vi "TDK_MsgManage.vi"(5 "CMD Type":T2=enum."SetADR", 6 "OUT?":bool, 7 "TDK Type":T1=enum."ZUP20-40", 8 "error in (no error)":errorcluster caption="error in", 9 "Current":dbl, 10 "Voltage":dbl, 11 "VISA resource name":refnum<visa-resource-name>) -> (0 "error out":errorcluster, 1 "Received Message":string, 3 "VISA resource name":refnum<visa-resource-name>, 4 "Serial Settings:Number of Bytes at Serial Port":u32)   [LabVIEW 2018]
uses:
  Def Ctrl/CMD Type.ctl
  Def Ctrl/TDK Type.ctl
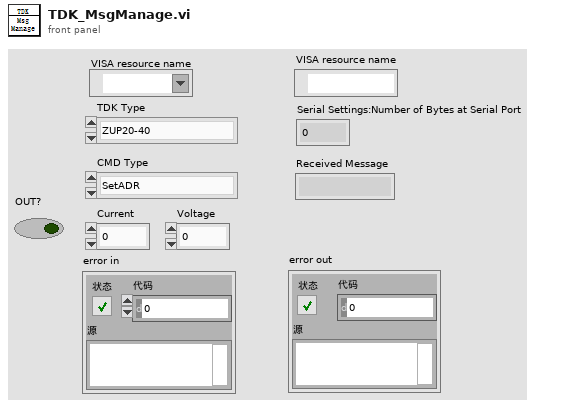
[diagram p1: front panel]
types:
  T1 = typedef "TDK Type.ctl" = enum16{"Default", "ZUP20-40", "Z+"}
  T2 = typedef "CMD Type.ctl" = enum16{"Default", "SetADR", "SetRMT", "SetVOL", "SetCUR", "SetOUT", "CheckREV", "CheckRMT", "CheckVOL", "CkeckCUR", "CheckOUT"}
  T3 = typedef "PowerSupplyCMD.ctl" = cluster{"ZUP20-40_CMD":T4, "Z+_CMD":T4}
  T4 = typedef "CMD_String.ctl" = cluster{"SetADR":string, "SetRMT":string, "SetVOL":string, "SetCUR":string, "SetOUT":string, "CheckREV":string, "CheckRMT":string, "CheckCUR":string, "CheckVOL":string, "CheckOUT":string}
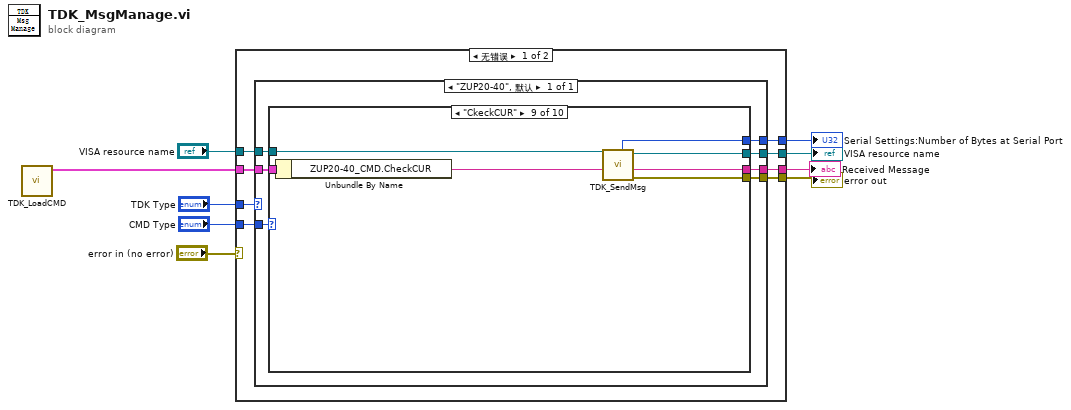
[diagram p0: block diagram]
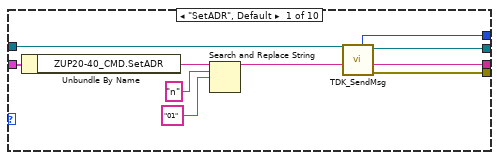
[diagram p2: hidden frame]
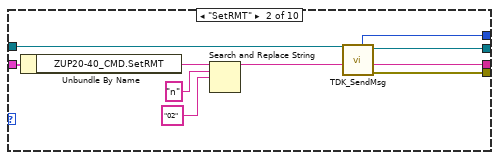
[diagram p3: hidden frame]
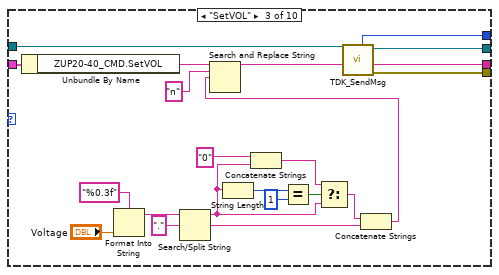
[diagram p4: hidden frame]
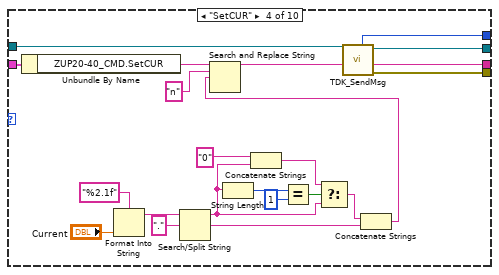
[diagram p5: hidden frame]
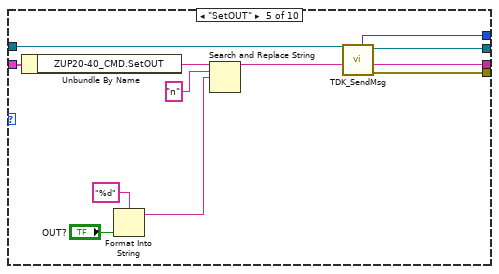
[diagram p6: hidden frame]
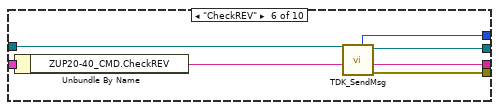
[diagram p7: hidden frame]
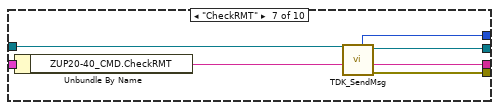
[diagram p8: hidden frame]
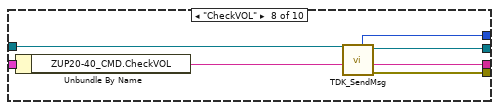
[diagram p9: hidden frame]
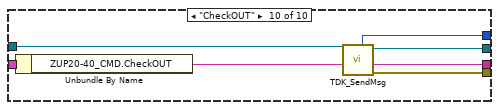
[diagram p10: hidden frame]
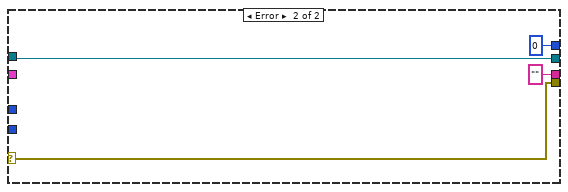
[diagram p11: hidden frame]
diagram:
  n1 = call "TDK_LoadCMD.vi"() -> ("PowerSupplyCMD"=w2:T3)  [unwired: 11 in]
  n2 = case shown="无错误" "error in (no error)" {
    selector: "error in (no error)" -> [_ w136]
    tunnel: "TDK Type" -> [w17 _]
    tunnel: "CMD Type" -> [w16 _]
    tunnel: "VISA resource name" -> [w15 w138]
    tunnel: [w14 u32 0 ("Serial Settings:Number of Bytes at Serial Port")] -> w6
    tunnel: [w13 w138] -> w5
    tunnel: [w12 "" ("Received Message")] -> w4
    tunnel: [w11 w136] -> w3
    tunnel: w2 -> [w10 _]
    frame No Error {
      n3 = case shown="\"ZUP20-40\", 默认" w17 {
        tunnel: w16 -> [w24]
        tunnel: w10 -> [w23]
        tunnel: w15 -> [w22]
        tunnel: [w21] -> w12
        tunnel: [w20] -> w13
        tunnel: [w19] -> w11
        tunnel: [w18] -> w14
        frame "ZUP20-40", Default {
          n4 = case shown="\"CkeckCUR\"" w24 {
            tunnel: w23 -> [w34 w44 w66 w88 w100 w107 w114 w121 w128 w135]
            tunnel: w22 -> [w33 w43 w65 w87 w99 w106 w113 w120 w127 w134]
            tunnel: [w28 w38 w61 w83 w95 w105 w112 w119 w126 w133] -> w21
            tunnel: [w27 w37 w60 w82 w94 w104 w111 w118 w125 w132] -> w20
            tunnel: [w26 w36 w59 w81 w93 w103 w110 w117 w124 w131] -> w19
            tunnel: [w25 w35 w58 w80 w92 w102 w109 w116 w123 w130] -> w18
            frame "SetADR", Default {
              n5 = Unbundle By Name(w34) -> ("ZUP20-40_CMD.SetADR"=w32:string)
              n6 = Search and Replace String(input string=w32, search string="n" ("搜索字符串"), replace string="01" ("替换字符串(\"\")")) -> (result string=w29:string)  [unwired: 5 in, 3 out]
              n7 = call "TDK_SendMsg.vi"("CMD"=w29, "VISA resource name"=w33) -> ("error out"=w26:errorcluster, "Received Message"=w28:string, "VISA resource name"=w27:refnum<visa-resource-name>, "Serial Settings:Number of Bytes at Serial Port"=w25:u32)  [unwired: 4 in]
            }
            frame "SetRMT" {
              n8 = Unbundle By Name(w44) -> ("ZUP20-40_CMD.SetRMT"=w42:string)
              n9 = Search and Replace String(input string=w42, search string="n" ("搜索字符串"), replace string="02" ("替换字符串(\"\")")) -> (result string=w39:string)  [unwired: 5 in, 3 out]
              n10 = call "TDK_SendMsg.vi"("CMD"=w39, "VISA resource name"=w43) -> ("error out"=w36:errorcluster, "Received Message"=w38:string, "VISA resource name"=w37:refnum<visa-resource-name>, "Serial Settings:Number of Bytes at Serial Port"=w35:u32)  [unwired: 4 in]
            }
            frame "SetVOL" {
              n11 = Unbundle By Name(w66) -> ("ZUP20-40_CMD.SetVOL"=w64:string)
              n12 = Format Into String(format string="%0.3f" ("Command Out"), "Voltage") -> (resulting string=w54:string)  [unwired: 2 in, 1 out]
              n13 = Search/Split String(string=w54, search string/char (-)=".") -> (substring before match=w48:string, match + rest of string=w46:string)  [unwired: 1 in, 1 out]
              n14 = String Length(string=w48) -> (length=w53:i32)
              n15 = Concatenate Strings("0" ("string"), w48) -> (w50:string)
              n16 = Equal?(x=w53, y=1) -> (x = y?=w51:bool)
              n17 = Select(t=w50, s=w51, f=w48) -> (s? t:f=w47:string)
              n18 = Concatenate Strings(w47, w46) -> (w45:string)
              n19 = Search and Replace String(input string=w64, search string="n" ("搜索字符串"), replace string=w45) -> (result string=w62:string)  [unwired: 5 in, 3 out]
              n20 = call "TDK_SendMsg.vi"("CMD"=w62, "VISA resource name"=w65) -> ("error out"=w59:errorcluster, "Received Message"=w61:string, "VISA resource name"=w60:refnum<visa-resource-name>, "Serial Settings:Number of Bytes at Serial Port"=w58:u32)  [unwired: 4 in]
            }
            frame "SetCUR" {
              n21 = Unbundle By Name(w88) -> ("ZUP20-40_CMD.SetCUR"=w86:string)
              n22 = Format Into String(format string="%2.1f" ("Command Out"), "Current") -> (resulting string=w76:string)  [unwired: 2 in, 1 out]
              n23 = Search/Split String(string=w76, search string/char (-)=".") -> (substring before match=w70:string, match + rest of string=w68:string)  [unwired: 1 in, 1 out]
              n24 = String Length(string=w70) -> (length=w75:i32)
              n25 = Concatenate Strings("0" ("string"), w70) -> (w72:string)
              n26 = Equal?(x=w75, y=1) -> (x = y?=w73:bool)
              n27 = Select(t=w72, s=w73, f=w70) -> (s? t:f=w69:string)
              n28 = Concatenate Strings(w69, w68) -> (w67:string)
              n29 = Search and Replace String(input string=w86, search string="n" ("搜索字符串"), replace string=w67) -> (result string=w84:string)  [unwired: 5 in, 3 out]
              n30 = call "TDK_SendMsg.vi"("CMD"=w84, "VISA resource name"=w87) -> ("error out"=w81:errorcluster, "Received Message"=w83:string, "VISA resource name"=w82:refnum<visa-resource-name>, "Serial Settings:Number of Bytes at Serial Port"=w80:u32)  [unwired: 4 in]
            }
            frame "SetOUT" {
              n31 = Unbundle By Name(w100) -> ("ZUP20-40_CMD.SetOUT"=w98:string)
              n32 = Format Into String(format string="%d" ("Command Out"), "OUT?") -> (resulting string=w89:string)  [unwired: 2 in, 1 out]
              n33 = Search and Replace String(input string=w98, search string="n" ("搜索字符串"), replace string=w89) -> (result string=w96:string)  [unwired: 5 in, 3 out]
              n34 = call "TDK_SendMsg.vi"("CMD"=w96, "VISA resource name"=w99) -> ("error out"=w93:errorcluster, "Received Message"=w95:string, "VISA resource name"=w94:refnum<visa-resource-name>, "Serial Settings:Number of Bytes at Serial Port"=w92:u32)  [unwired: 4 in]
            }
            frame "CheckREV" {
              n35 = Unbundle By Name(w107) -> ("ZUP20-40_CMD.CheckREV"=w101:string)
              n36 = call "TDK_SendMsg.vi"("CMD"=w101, "VISA resource name"=w106) -> ("error out"=w103:errorcluster, "Received Message"=w105:string, "VISA resource name"=w104:refnum<visa-resource-name>, "Serial Settings:Number of Bytes at Serial Port"=w102:u32)  [unwired: 4 in]
            }
            frame "CheckRMT" {
              n37 = Unbundle By Name(w114) -> ("ZUP20-40_CMD.CheckRMT"=w108:string)
              n38 = call "TDK_SendMsg.vi"("CMD"=w108, "VISA resource name"=w113) -> ("error out"=w110:errorcluster, "Received Message"=w112:string, "VISA resource name"=w111:refnum<visa-resource-name>, "Serial Settings:Number of Bytes at Serial Port"=w109:u32)  [unwired: 4 in]
            }
            frame "CheckVOL" {
              n39 = Unbundle By Name(w121) -> ("ZUP20-40_CMD.CheckVOL"=w115:string)
              n40 = call "TDK_SendMsg.vi"("CMD"=w115, "VISA resource name"=w120) -> ("error out"=w117:errorcluster, "Received Message"=w119:string, "VISA resource name"=w118:refnum<visa-resource-name>, "Serial Settings:Number of Bytes at Serial Port"=w116:u32)  [unwired: 4 in]
            }
            frame "CkeckCUR" {
              n41 = Unbundle By Name(w128) -> ("ZUP20-40_CMD.CheckCUR"=w122:string)
              n42 = call "TDK_SendMsg.vi"("CMD"=w122, "VISA resource name"=w127) -> ("error out"=w124:errorcluster, "Received Message"=w126:string, "VISA resource name"=w125:refnum<visa-resource-name>, "Serial Settings:Number of Bytes at Serial Port"=w123:u32)  [unwired: 4 in]
            }
            frame "CheckOUT" {
              n43 = Unbundle By Name(w135) -> ("ZUP20-40_CMD.CheckOUT"=w129:string)
              n44 = call "TDK_SendMsg.vi"("CMD"=w129, "VISA resource name"=w134) -> ("error out"=w131:errorcluster, "Received Message"=w133:string, "VISA resource name"=w132:refnum<visa-resource-name>, "Serial Settings:Number of Bytes at Serial Port"=w130:u32)  [unwired: 4 in]
            }
          }
        }
      }
    }
    frame Error {
    }
  }
  "Serial Settings:Number of Bytes at Serial Port" <- w6
  "VISA resource name" <- w5
  "Received Message" <- w4
  "error out" <- w3
